vi "Lasing-handler.vi"(8 "error in (no error)":errorcluster, 11 "Object ref in":T1) -> (0 "error out":errorcluster, 3 "Object ref out":T1)   [LabVIEW 2013, in "SLMControl.lvlib" / "SC-Main.lvclass"]
uses:
  SC-Main.lvclass
  Object-reference.ctl
  Lasing-actions.ctl
  Main-actions.ctl
  Enqueue-modes.ctl
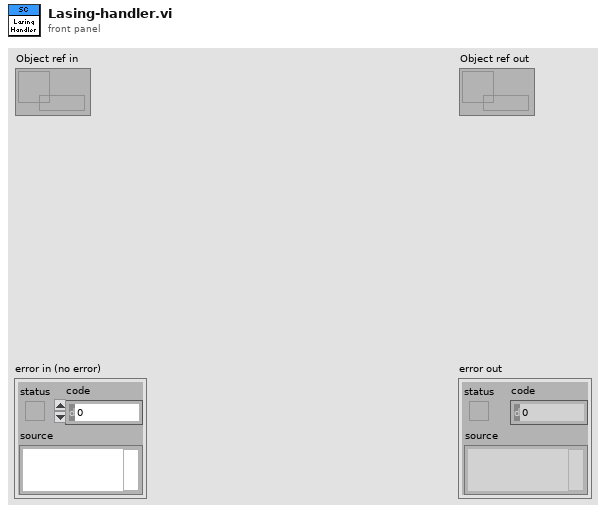
[diagram p1: front panel]
types:
  T1 = typedef "SLMControl.lvlib/SC-Main.lvclass/Object-reference.ctl" = refnum<data-value>
  T2 = typedef "SLMControl.lvlib/SC-Main.lvclass/Lasing-actions.ctl" = enum16{"Idle", "Activate", "Load lasing file", "Launch lasing", "Wait for lasing end", "Signal iterate", "Signal abort", "Abort", "Reset", "Exit"}
  T3 = typedef "SLMControl.lvlib/SC-Main.lvclass/Enqueue-modes.ctl" = enum16{"Default", "Priority", "Flush"}
  T4 = typedef "SLMControl.lvlib/SC-Main.lvclass/Main-actions.ctl" = enum16{"Idle", "Initialize", "Load configuration", "Save configuration", "Load lasing files", "Load deposition files", "Refresh files", "Clear files", "Open lasing file", "Activate", "Start", "Start deposition cycle", "Start lasing cycle", "Iterate", "Abort", "Stop", "Exit"}
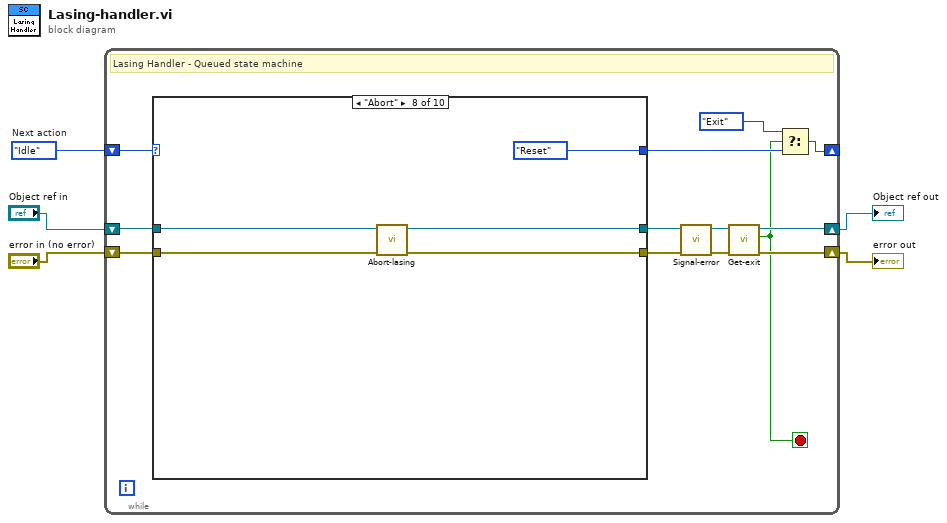
[diagram p0: block diagram]
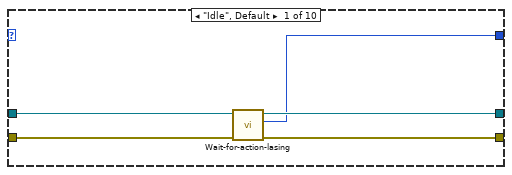
[diagram p2: hidden frame]
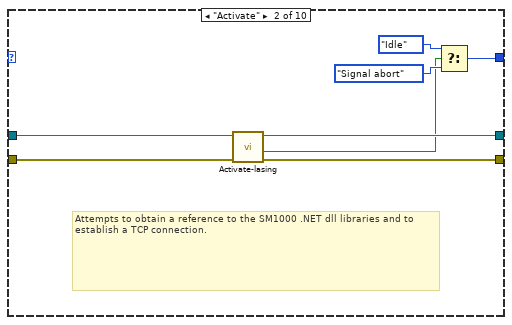
[diagram p3: hidden frame]
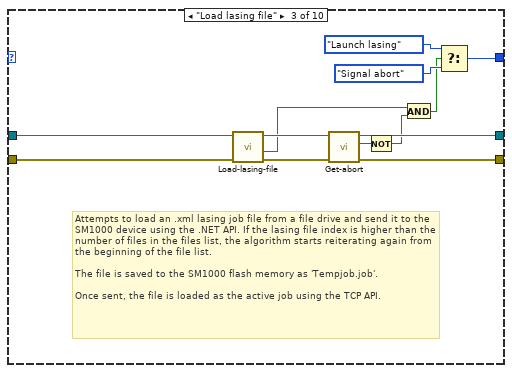
[diagram p4: hidden frame]
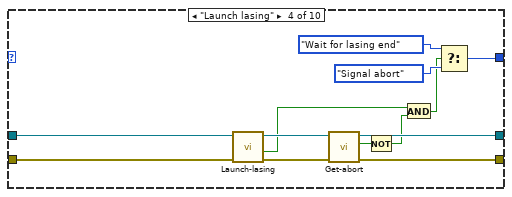
[diagram p5: hidden frame]
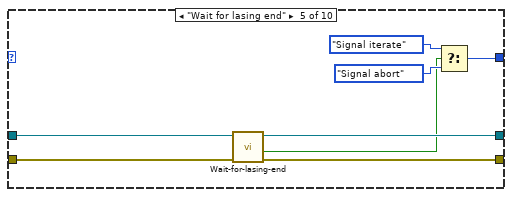
[diagram p6: hidden frame]
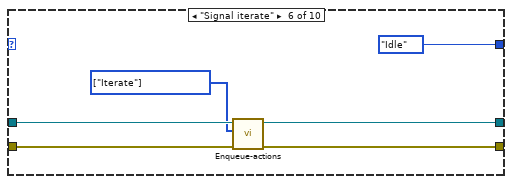
[diagram p7: hidden frame]
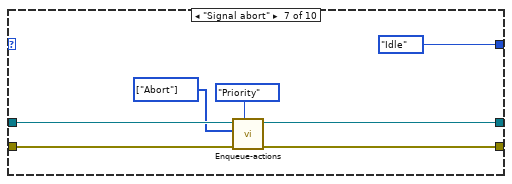
[diagram p8: hidden frame]
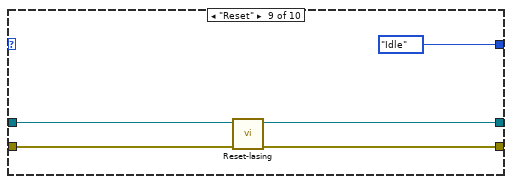
[diagram p9: hidden frame]
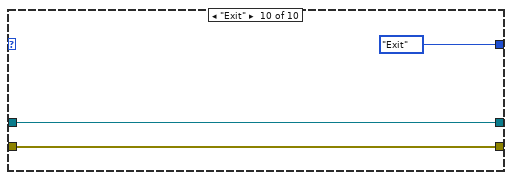
[diagram p10: hidden frame]
diagram:
  w5 = Lasing-actions."Idle"  # Next action
  n1 = while {
    shift-right: [w10] -> _
    shift-left: w5 -> [w18]
    shift-right: [w8] -> w4
    shift-left: "error in (no error)" -> [w17]
    shift-right: [w13] -> w3
    shift-left: "Object ref in" -> [w16]
    stop <- w6 stop-if-true
    # "Lasing Handler - Queued state machine"
    n2 = case shown="\"Abort\"" w18 {
      tunnel: w17 -> [w19 w30 w43 w56 w64 w69 w76 w81 w86 w89]
      tunnel: [w21 w28 w35 w48 w59 w66 w72 w79 w84 w89] -> w7
      tunnel: [w20 w25 w42 w53 w63 Lasing-actions."Idle" ("Action Handler states") Lasing-actions."Idle" ("Action Handler states") Lasing-actions."Reset" ("Action Handler states") Lasing-actions."Idle" ("Action Handler states") Lasing-actions."Exit" ("Action Handler states")] -> w11
      tunnel: w16 -> [w23 w31 w44 w57 w65 w70 w77 w82 w87 w90]
      tunnel: [w22 w29 w36 w49 w60 w67 w73 w80 w85 w90] -> w15
      frame "Idle", Default {
        n3 = call "Wait-for-action-lasing.vi"("error in (no error)"=w19, "Object ref in"=w23) -> ("error out"=w21:errorcluster, "Action"=w20:T2, "Object ref out"=w22:T1)  [unwired: 7 in]
      }
      frame "Activate" {
        # "Attempts to obtain a reference to the SM1000 .NET dll libraries and to establish a TCP connection."
        n4 = call "Activate-lasing.vi"("error in (no error)"=w30, "Object ref in"=w31) -> ("error out"=w28:errorcluster, "Succes?"=w24:bool, "Object ref out"=w29:T1)  [unwired: 7 in]
        n5 = Select(t=Lasing-actions."Idle" ("Action Handler states"), s=w24, f=Lasing-actions."Signal abort" ("Action Handler states")) -> (s? t:f=w25:T2)
      }
      frame "Load lasing file" {
        # "Attempts to load an .xml lasing job file from a file drive and send it to the SM1000 device using the .NET API. If the lasing file index is higher than the number of files in the files list, the algorithm starts reiterating again from the beginning of the file list.\n\nThe file is saved to the SM1000 flash memory as 'Tempjob.job'.\n\nOnce sent, the file is loaded as the active job using the TCP API."
        n6 = call "Load-lasing-file.vi"("error in (no error)"=w43, "Object ref in"=w44) -> ("error out"=w37:errorcluster, "Succes?"=w34:bool, "Object ref out"=w38:T1)  [unwired: 7 in]
        n7 = call "Get-abort.vi"("error in (no error)"=w37, "Object ref in"=w38) -> ("error out"=w35:errorcluster, "Abort"=w39:bool, "Object ref out"=w36:T1)  [unwired: 7 in]
        n8 = Not(x=w39) -> (.not. x?=w33:bool)
        n9 = And(x=w34, y=w33) -> (x .and. y?=w32:bool)
        n10 = Select(t=Lasing-actions."Launch lasing" ("Action Handler states"), s=w32, f=Lasing-actions."Signal abort" ("Action Handler states")) -> (s? t:f=w42:T2)
      }
      frame "Launch lasing" {
        n11 = call "Launch-lasing.vi"("error in (no error)"=w56, "Object ref in"=w57) -> ("error out"=w54:errorcluster, "Succes?"=w45:bool, "Object ref out"=w55:T1)  [unwired: 7 in]
        n12 = call "Get-abort.vi"("error in (no error)"=w54, "Object ref in"=w55) -> ("error out"=w48:errorcluster, "Abort"=w50:bool, "Object ref out"=w49:T1)  [unwired: 7 in]
        n13 = Not(x=w50) -> (.not. x?=w47:bool)
        n14 = And(x=w45, y=w47) -> (x .and. y?=w46:bool)
        n15 = Select(t=Lasing-actions."Wait for lasing end" ("Action Handler states"), s=w46, f=Lasing-actions."Signal abort" ("Action Handler states")) -> (s? t:f=w53:T2)
      }
      frame "Wait for lasing end" {
        n16 = call "Wait-for-lasing-end.vi"("error in (no error)"=w64, "Object ref in"=w65) -> ("error out"=w59:errorcluster, "Succes?"=w58:bool, "Object ref out"=w60:T1)  [unwired: 7 in]
        n17 = Select(t=Lasing-actions."Signal iterate" ("Action Handler states"), s=w58, f=Lasing-actions."Signal abort" ("Action Handler states")) -> (s? t:f=w63:T2)
      }
      frame "Signal iterate" {
        w68 = T4[] [enum."Iterate"] items=["Idle", "Initialize", "Load configuration", "Save configuration", "Load lasing files", "Load deposition files", "Refresh files", "Clear files", "Open lasing file", "Activate", "Start", "Start deposition cycle", "Start lasing cycle", "Iterate", "Abort", "Stop", "Exit"] ("State array")
        n18 = call "Enqueue-actions.vi"("error in (no error)"=w69, "State array"=w68, "State queue in"=w70) -> ("error out"=w66:errorcluster, "State queue out"=w67:T1)  [unwired: 6 in, 1 out]
      }
      frame "Signal abort" {
        w74 = T4[] [enum."Abort"] items=["Idle", "Initialize", "Load configuration", "Save configuration", "Load lasing files", "Load deposition files", "Refresh files", "Clear files", "Open lasing file", "Activate", "Start", "Start deposition cycle", "Start lasing cycle", "Iterate", "Abort", "Stop", "Exit"] ("State array")
        n19 = call "Enqueue-actions.vi"("Enqueue mode"=Enqueue-modes."Priority", "error in (no error)"=w76, "State array"=w74, "State queue in"=w77) -> ("error out"=w72:errorcluster, "State queue out"=w73:T1)  [unwired: 5 in, 1 out]
      }
      frame "Abort" {
        n20 = call "Abort-lasing.vi"("error in (no error)"=w81, "Object ref in"=w82) -> ("error out"=w79:errorcluster, "Object ref out"=w80:T1)  [unwired: 8 in]
      }
      frame "Reset" {
        n21 = call "Reset-lasing.vi"("error in (no error)"=w86, "Object ref in"=w87) -> ("error out"=w84:errorcluster, "Object ref out"=w85:T1)  [unwired: 8 in]
      }
      frame "Exit" {
      }
    }
    n22 = call "Signal-error.vi"("error in (no error)"=w7, "Data in"=w15) -> ("error out"=w12:errorcluster, "Data out"=w14:T1)  [unwired: 8 in]
    n23 = call "Get-exit.vi"("error in (no error)"=w12, "Object ref in"=w14) -> ("error out"=w8:errorcluster, "Exit?"=w6:bool, "Object ref out"=w13:T1)  [unwired: 7 in]
    n24 = Select(t=Lasing-actions."Exit", s=w6, f=w11) -> (s? t:f=w10:T2)
  }
  "error out" <- w4
  "Object ref out" <- w3
